vi "GetSpeedProfileDataSetProps.vi"(6 "do not write to database":bool, 8 "error in (no error)":errorcluster, 11 "dataset props in":T1[](array[typedef])) -> (0 "error out":errorcluster, 3 "dataset props out":T1[](array[typedef]))   [LabVIEW 2017, in "CmsDataEventCreator.lvlib"]
uses:
  <vilib>/addons/InsightCM/Devices/Shared/Cms/CmsDataEventCreator/CmsDataEventCreator.lvlib
  <vilib>/addons/InsightCM/MessageBus/Base/controls/KeyValuePair.ctl
  <vilib>/addons/InsightCM/Utilities/PropertyHelpers/PropertyHelpers.lvlib
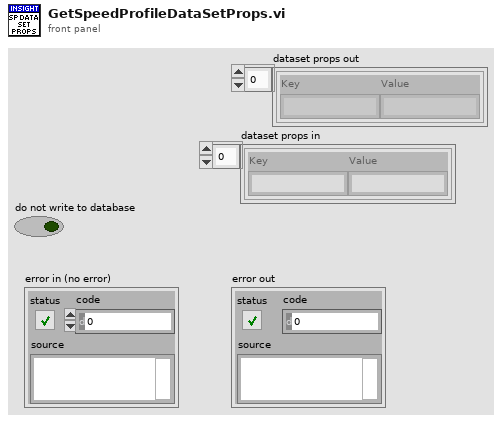
[diagram p1: front panel]
types:
  T1 = typedef "KeyValuePair.ctl" = cluster{"Key":string, "Value":string}
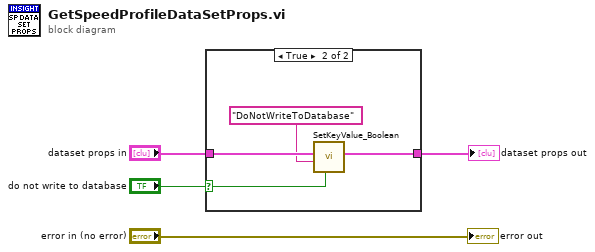
[diagram p0: block diagram]
diagram:
  n1 = case shown="True" "do not write to database" {
    selector: "do not write to database" -> [_ w6]
    tunnel: "dataset props in" -> [w5 w9]
    tunnel: [w5 w8] -> w4
    frame False {
    }
    frame True {
      n2 = call <vilib>:"SetKeyValue_Boolean.vi"("value"=w6, "key"="DoNotWriteToDatabase", "key value pairs"=w9) -> ("key value pairs out"=w8:T1[])  [unwired: 8 in]
    }
  }
  "dataset props out" <- w4
  "error out" <- "error in (no error)"
